vi "Render.vi"(8 "error in":errorcluster, 10 "Renderer in":refnum<class "Renderer.lvclass">, 11 "object in":refnum<class "TAFConfiguration.lvclass">) -> (0 "error out":errorcluster, 3 "Sections out":refnum<class "Section.lvclass">[](array[class]))   [LabVIEW 2021, in "TAF Proj Document Type.lvlib" / "TAFConfiguration.lvclass"]
uses:
  <vilib>/Wovalab/AntiDoc/Document Type/Add-ons/LabVIEW TAF Project/TAFConfiguration/TAFConfiguration.lvclass
  C:/Program Files (x86)/National Instruments/LabVIEW 2021/vi.lib/Wovalab/AntiDoc/Bloc/Bloc.lvclass
  <vilib>/Wovalab/AsciiDoc for LabVIEW/Section/Section.lvclass
  <vilib>/Wovalab/AntiDoc/Renderer/Renderer.lvclass
  <vilib>/Wovalab/AntiDoc/Document Type/Add-ons/LabVIEW TAF Project/TAFConfiguration/TAFConfiguration.lvclass/TAFConfiguration.ctl
  <vilib>/Wovalab/AsciiDoc for LabVIEW/Diagram/Type--enum.ctl
  <vilib>/Wovalab/AntiDoc/Bloc/Bloc.lvclass/Bloc.ctl
  <vilib>/Wovalab/AsciiDoc for LabVIEW/Table/Table.lvclass/Table.ctl
  <vilib>/Wovalab/AntiDoc/Bloc/Read Name.vi
  <vilib>/Wovalab/AsciiDoc for LabVIEW/Table/Table.lvclass
  C:/Program Files (x86)/National Instruments/LabVIEW 2021/vi.lib/Wovalab/AsciiDoc for LabVIEW/Adoc-Bloc/Bloc.lvclass
  <vilib>/Wovalab/AsciiDoc for LabVIEW/Diagram/Diagram.lvclass
  <vilib>/Wovalab/AsciiDoc for LabVIEW/Paragraph/Paragraph.lvclass
  <vilib>/Wovalab/AsciiDoc for LabVIEW/Sub Section/Sub Section.lvclass
  C:/Program Files (x86)/National Instruments/LabVIEW 2021/vi.lib/Wovalab/AsciiDoc for LabVIEW/Section/Section.lvclass
  <vilib>/Wovalab/AsciiDoc for LabVIEW/Section/Add Bloc (scalar).vi
  <vilib>/Wovalab/AsciiDoc for LabVIEW/Sub Section/Create Sub Section (array).vi
  <vilib>/Wovalab/AsciiDoc for LabVIEW/Sub Section/Create Sub Section (scalar).vi
  <vilib>/Wovalab/AsciiDoc for LabVIEW/Section/Add Bloc (array).vi
  <vilib>/Wovalab/AntiDoc/Utilities/Utilities.lvlib
  <vilib>/Wovalab/AntiDoc/Document Type/Add-ons/LabVIEW TAF Project/TAF Proj Document Type.lvlib
  C:/Program Files (x86)/National Instruments/LabVIEW 2021/vi.lib/Wovalab/AsciiDoc for LabVIEW/Table/Table.lvclass
  C:/Program Files (x86)/National Instruments/LabVIEW 2021/vi.lib/Wovalab/AsciiDoc for LabVIEW/Paragraph/Paragraph.lvclass
  C:/Program Files (x86)/National Instruments/LabVIEW 2021/vi.lib/Wovalab/AsciiDoc for LabVIEW/Diagram/Diagram.lvclass
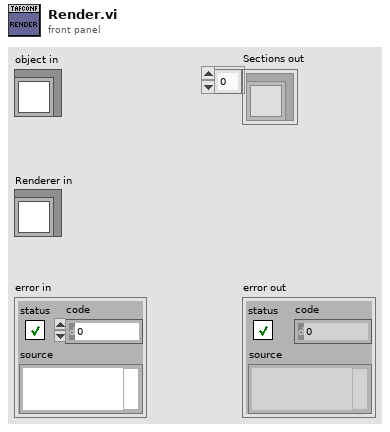
[diagram p1: front panel]
types:
  T1 = cluster{"ObjectName":string, "ObjectType":string, "Interfaces":cluster{"Label":string, "ObjectName":string, "Type":string}[]}[]
  T2 = cluster{"ObjectName":string, "ObjectFile":string, "FileContent":string}[]
  T3 = cluster{"Captions":string[], "EnablesExpressions":string[], "ActionTypes":string[], "TargetObjects":string[], "Parameters":string[]}
  T4 = typedef "Wovalab_lib_AsciiDoctor.lvlib/Diagram.lvclass/Type--enum.ctl" = enum16{"a2s", "actdiag", "blockdiag", "ditaa", "erd", "graphviz", "meme", "mermaid", "msc", "nwdiag", "packetdiag", "plantuml", "rackdiag", "seqdiag", "shaape", "svgbob", "syntrax", "umlet", "vega", "vegalite", "wavedrom"}
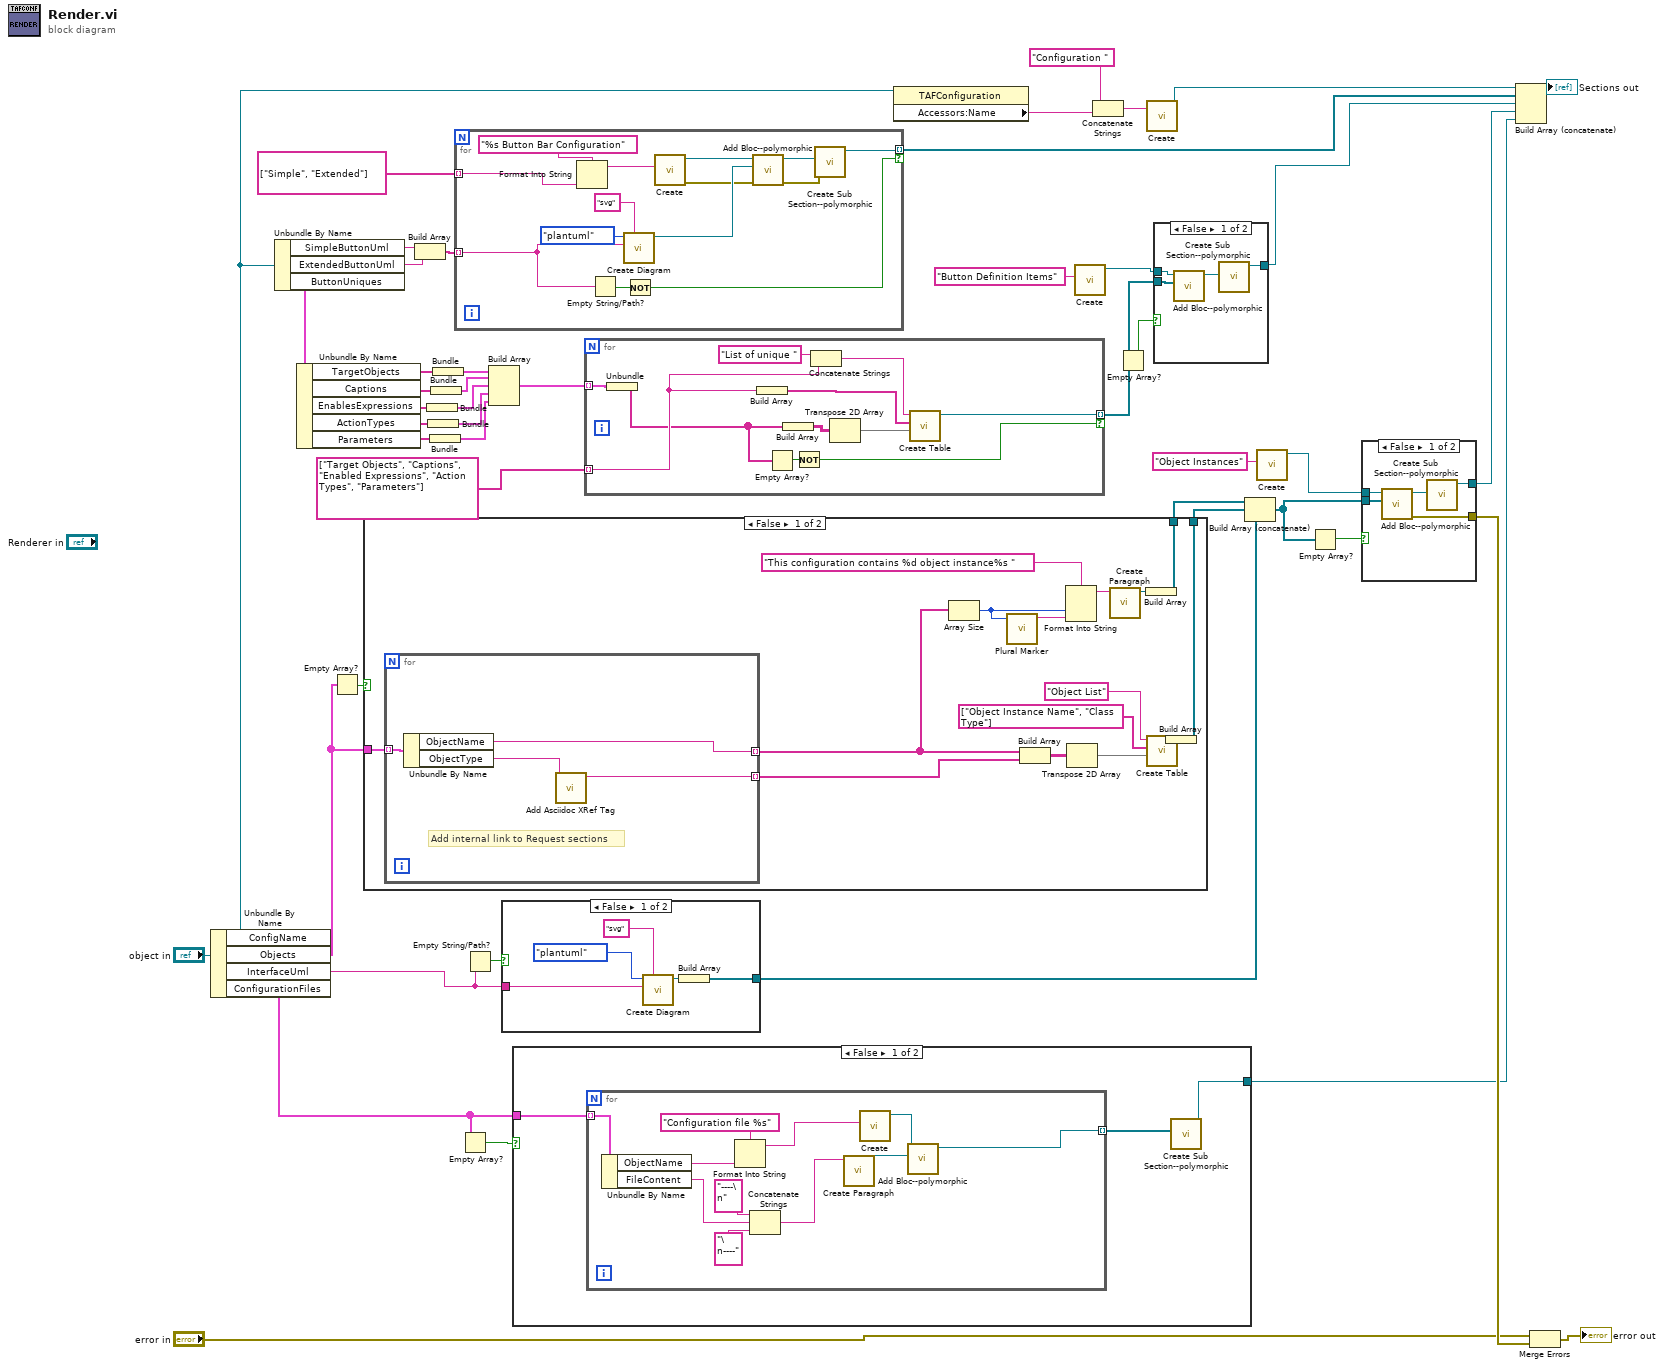
[diagram p0: block diagram]
diagram:
  n1 = Unbundle By Name("object in") -> ("Objects"=w26:T1, "InterfaceUml"=w24:string, "ConfigurationFiles"=w2:T2)  [unwired: 1 out]
  n2 = Unbundle By Name("object in") -> ("SimpleButtonUml"=w36:string, "ExtendedButtonUml"=w35:string, "ButtonUniques"=w21:T3)
  n3 = Unbundle By Name(w21) -> ("TargetObjects"=w20:string[], "Captions"=w19:string[], "EnablesExpressions"=w18:string[], "ActionTypes"=w17:string[], "Parameters"=w16:string[])
  n4 = Empty Array?(array=w26) -> (empty?=w27:bool)
  n5 = case shown="False" w27 {
    tunnel: w26 -> [w52 _]
    tunnel: [w49 _] -> w41
    tunnel: [w48 _] -> w40
    frame False {
      n6 = for {
        tunnel: [w64] -> w58 mode=indexing
        tunnel: [w63] -> w55 mode=indexing
        tunnel: w52 -> [w66] mode=indexing
        # "Add internal link to Request sections"
        n7 = Unbundle By Name(w66) -> ("ObjectName"=w64:string, "ObjectType"=w65:string)
        n8 = call <vilib>:"Add Asciidoc XRef Tag.vi"("String In"=w65) -> ("String out"=w63:string)  [unwired: 10 in]
      }
      n9 = Array Size(array=w58) -> (size(s)=w54:i32)
      n10 = call <vilib>:"Plural Marker.vi"("Size"=w54) -> ("Plural Mark"=w53:string)  [unwired: 10 in]
      n11 = Build Array(w58, w55) -> (w60:string[][])
      n12 = Format Into String(format string="This configuration contains %d object instance%s " ("Content"), w54, w53) -> (resulting string=w57:string)  [unwired: 2 in, 1 out]
      n13 = Transpose 2D Array(2D array=w60) -> (transposed array=w59:string[][])
      n14 = call <vilib>:"Create Paragraph.vi"("Content"=w57) -> ("Paragraph out"=w51:refnum<class "Paragraph.lvclass">)  [unwired: 9 in, 1 out]
      n15 = Build Array(w51) -> (w49:refnum<class "Paragraph.lvclass">[])
      n16 = call <vilib>:"Create Table.vi"("Content"=w59, "Header"=string[] ["Object Instance Name", "Class Type"], "Title"="Object List") -> ("Table out"=w50:refnum<class "Table.lvclass">)  [unwired: 7 in, 1 out]
      n17 = Build Array(w50) -> (w48:refnum<class "Table.lvclass">[])
    }
    frame True {
    }
  }
  n18 = Build Array(w36, w35) -> (w34:string[])
  n19 = Bundle("EnablesExpressions"=w18) -> (w13:cluster{"EnablesExpressions":string[]})  [unwired: 1 in]
  n20 = Bundle("ActionTypes"=w17) -> (w12:cluster{"ActionTypes":string[]})  [unwired: 1 in]
  n21 = Bundle("Parameters"=w16) -> (w11:cluster{"Parameters":string[]})  [unwired: 1 in]
  n22 = Bundle("Captions"=w19) -> (w14:cluster{"Captions":string[]})  [unwired: 1 in]
  n23 = Bundle("TargetObjects"=w20) -> (w15:cluster{"TargetObjects":string[]})  [unwired: 1 in]
  n24 = for {
    tunnel: w34 -> [w69] mode=indexing
    tunnel: string[] ["Simple", "Extended"] ("appended array") -> [w77] mode=indexing
    tunnel: [w70] -> w29 mode=indexing if=w67
    n25 = Format Into String(format string="%s Button Bar Configuration" ("Content"), w77) -> (resulting string=w76:string)  [unwired: 2 in, 1 out]
    n26 = Empty String/Path?(string/path=w69) -> (empty?=w68:bool)
    n27 = call <vilib>:"Create Diagram.vi"("Format (png)"="svg", "Diagram Source Code"=w69, "Diagram Type"=Type--enum."plantuml") -> ("Diagram out"=w75:refnum<class "Diagram.lvclass">)  [unwired: 7 in, 1 out]
    n28 = Not(x=w68) -> (.not. x?=w67:bool)
    n29 = call <vilib>:"Create.vi"("Title"=w76) -> ("error out"=w74:errorcluster, "Section out"=w72:refnum<class "Section.lvclass">)  [unwired: 9 in]
    n30 = call-poly <vilib>:"Add Bloc--polymorphic.vi"("error in"=w74, "Bloc"=w75, "Section in"=w72) -> ("error out"=w73:errorcluster, "Section out"=w71:refnum<class "Section.lvclass">)  [unwired: 7 in]
    n31 = call-poly <vilib>:"Create Sub Section--polymorphic.vi"("error in (no error)"=w73, "Section"=w71) -> ("Sub Section out"=w70:refnum<class "Sub Section.lvclass">)  [unwired: 8 in, 1 out]
  }
  n32 = Empty Array?(array=w2) -> (empty?=w3:bool)
  n33 = Empty String/Path?(string/path=w24) -> (empty?=w25:bool)
  n34 = Build Array(w15, w14, w13, w12, w11) -> (w10:cluster{"Parameters":string[]}[])
  n35 = case shown="False" w25 {
    tunnel: [w81 _] -> w45
    tunnel: w24 -> [w82 _]
    frame False {
      n36 = call <vilib>:"Create Diagram.vi"("Format (png)"="svg", "Diagram Source Code"=w82, "Diagram Type"=Type--enum."plantuml") -> ("Diagram out"=w84:refnum<class "Diagram.lvclass">)  [unwired: 7 in, 1 out]
      n37 = Build Array(w84) -> (w81:refnum<class "Diagram.lvclass">[])
    }
    frame True {
    }
  }
  n38 = case shown="False" w3 {
    tunnel: w2 -> [w88 _]
    tunnel: [w86 _] -> w1
    frame False {
      n39 = for {
        tunnel: w88 -> [w99] mode=indexing
        tunnel: [w93] -> w87 mode=indexing
        n40 = Unbundle By Name(w99) -> ("ObjectName"=w96:string, "FileContent"=w90:string)
        n41 = Format Into String(format string="Configuration file %s" ("Title"), w96) -> (resulting string=w95:string)  [unwired: 2 in, 1 out]
        n42 = Concatenate Strings("----\n" ("string"), w90, "\n----" ("string")) -> (w92:string)
        n43 = call <vilib>:"Create Paragraph.vi"("Content"=w92) -> ("Paragraph out"=w94:refnum<class "Paragraph.lvclass">)  [unwired: 9 in, 1 out]
        n44 = call <vilib>:"Create.vi"("Title"=w95) -> ("Section out"=w98:refnum<class "Section.lvclass">)  [unwired: 9 in, 1 out]
        n45 = call-poly <vilib>:"Add Bloc--polymorphic.vi"("Bloc"=w94, "Section in"=w98) -> ("Section out"=w93:refnum<class "Section.lvclass">)  [unwired: 8 in, 1 out]
      }
      n46 = call-poly <vilib>:"Create Sub Section--polymorphic.vi"("Section"=w87) -> ("Sub Section out"=w86:refnum<class "Sub Section.lvclass">)  [unwired: 9 in, 1 out]
    }
    frame True {
    }
  }
  n47 = for {
    tunnel: w10 -> [w110] mode=indexing
    tunnel: string[] ["Target Objects", "Captions", "Enabled Expressions", "Action Types", "Parameters"] -> [w105] mode=indexing
    tunnel: [w103] -> w5 mode=indexing if=w100
    n48 = Unbundle(w110) -> ("Parameters"=w102:string[])
    n49 = Build Array(w105) -> (w104:string[])
    n50 = Empty Array?(array=w102) -> (empty?=w101:bool)
    n51 = Build Array(w102) -> (w108:string[][])
    n52 = Not(x=w101) -> (.not. x?=w100:bool)
    n53 = Concatenate Strings("List of unique " ("string"), w105) -> (w107:string)
    n54 = Transpose 2D Array(2D array=w108) -> (transposed array=w109:string[][])
    n55 = call <vilib>:"Create Table.vi"("Content"=w109, "Header"=w104, "Title"=w107) -> ("Table out"=w103:refnum<class "Table.lvclass">)  [unwired: 7 in, 1 out]
  }
  n56 = property class="TAFConfiguration"(reference="object in") -> ("Accessors:Name"=w44:string)  [unwired: 1 in, 2 out]
  n57 = call <vilib>:"Create.vi"("Title"="Button Definition Items") -> ("Section out"=w6:refnum<class "Section.lvclass">)  [unwired: 9 in, 1 out]
  n58 = Concatenate Strings("Configuration " ("Content"), w44) -> (w39:string)
  n59 = Empty Array?(array=w5) -> (empty?=w7:bool)
  n60 = call <vilib>:"Create.vi"("Title"=w39) -> ("Section out"=w30:refnum<class "Section.lvclass">)  [unwired: 9 in, 1 out]
  n61 = case shown="False" w7 {
    tunnel: w6 -> [w114 _]
    tunnel: [w112 _] -> w4
    tunnel: w5 -> [w111 _]
    frame False {
      n62 = call-poly <vilib>:"Add Bloc--polymorphic.vi"("Bloc"=w111, "Section in"=w114) -> ("Section out"=w113:refnum<class "Section.lvclass">)  [unwired: 8 in, 1 out]
      n63 = call-poly <vilib>:"Create Sub Section--polymorphic.vi"("Section"=w113) -> ("Sub Section out"=w112:refnum<class "Sub Section.lvclass">)  [unwired: 9 in, 1 out]
    }
    frame True {
    }
  }
  n64 = Build Array (concatenate)(w41, w40, w45) -> (w22:refnum<class "Bloc.lvclass">[])
  n65 = call <vilib>:"Create.vi"("Title"="Object Instances") -> ("Section out"=w32:refnum<class "Section.lvclass">)  [unwired: 9 in, 1 out]
  n66 = Empty Array?(array=w22) -> (empty?=w23:bool)
  n67 = case shown="False" w23 {
    tunnel: [w119 _] -> w46
    tunnel: w22 -> [w118 _]
    tunnel: w32 -> [w117 _]
    tunnel: [w115 _] -> w28
    frame False {
      n68 = call-poly <vilib>:"Add Bloc--polymorphic.vi"("Bloc"=w118, "Section in"=w117) -> ("error out"=w119:errorcluster, "Section out"=w116:refnum<class "Section.lvclass">)  [unwired: 8 in]
      n69 = call-poly <vilib>:"Create Sub Section--polymorphic.vi"("Section"=w116) -> ("Sub Section out"=w115:refnum<class "Sub Section.lvclass">)  [unwired: 9 in, 1 out]
    }
    frame True {
    }
  }
  n70 = Build Array (concatenate)(w30, w29, w4, w28, w1) -> (→"Sections out":refnum<class "Section.lvclass">[])
  n71 = Merge Errors("error in", w46) -> (→"error out":errorcluster)
